vi "Configure Sample Rate [ARB].vi"(8 "error in (no error)":errorcluster, 9 "sample rate (1000 Samp/s)":dbl[unit]=1000.0 format="%^.2e", 11 "CS++Fgen in":refnum<class "CS++Fgen.lvclass">) -> (0 "error out":errorcluster, 3 "CS++Fgen out":refnum<class "CS++Fgen.lvclass">)   [LabVIEW 2013, in "CS++Fgen.lvlib" / "CS++Fgen.lvclass"]
doc: "This VI configures the rate at which the function generator produces the points that make up arbitrary waveforms. When you configure the function generator to produce an arbitrary sequence, this is the sample rate for all arbitrary waveforms in the sequence.\n \nNotes:\n\n(1) This VI is part of the IviFgenArbWfm [ARB] extension group."
uses:
  CS++Fgen.lvclass
  Core/Classes/CS++ProcessVariables/ProcessVariable/PV.lvclass
  Core/Classes/CS++ProcessVariables/ProcessVariable/PV.lvclass/PV.ctl
  CS++Fgen.lvclass/CS++Fgen.ctl
  Core/Classes/CS++ProcessVariables/PVConnection/PVConnection.lvclass
  Core/Classes/CS++ProcessVariables/ProcessVariable/Write Data.vi
  Core/Classes/CS++ProcessVariables/ProcessVariable/Write Timestamp.vi
  Core/Classes/CS++ProcessVariables/ProcessVariable/Write Quality.vi
  Core/Classes/CS++ProcessVariables/ProcessVariable/Write status.vi
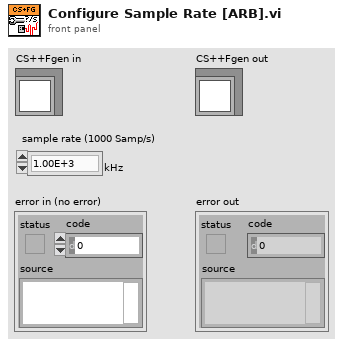
[diagram p1: front panel]
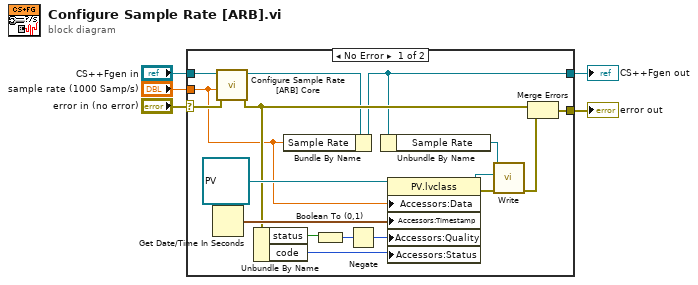
[diagram p0: block diagram]
diagram:
  n1 = case shown="No Error" "error in (no error)" {
    selector: "error in (no error)" -> [w21 w24]
    tunnel: [w10 w24] -> w4
    tunnel: [w6 w23] -> w2
    tunnel: "CS++Fgen in" -> [w22 w23]
    tunnel: "sample rate (1000 Samp/s)" -> [w8 _]
    frame No Error {
      n2 = Get Date/Time In Seconds() -> (seconds since 1Jan1904=w20:timestamp)
      n3 = call-dynamic "Configure Sample Rate [ARB] Core.vi"("error in (no error)"=w21, "sample rate (1000 Samp/s)"=w8, "CS++Fgen in"=w22) -> ("error out"=w9:errorcluster, "CS++Fgen out"=w7:refnum<class "CS++Fgen.lvclass">)  [unwired: 7 in]
      n4 = Unbundle By Name(w9) -> ("status"=w15:bool, "code"=w13:i32)
      n5 = Bundle By Name(cluster=w7, "Sample Rate"=w8) -> (w6:refnum<class "CS++Fgen.lvclass">)
      n6 = Boolean To (0,1)(Boolean=w15) -> (0, 1=w14:i16)
      n7 = Negate(x=w14) -> (-x=w12:i16)
      n8 = Unbundle By Name(w6) -> ("Sample Rate"=w11:refnum<class "PVConnection.lvclass">)
      n9 = property class="PV.lvclass"(reference=refnum<class "PV.lvclass"> refnum ("PV"), "Accessors:Data"=w8, "Accessors:Timestamp"=w20, "Accessors:Quality"=w12, "Accessors:Status"=w13) -> (reference out=w17:refnum<class "PV.lvclass">, error out=w18:errorcluster)  [unwired: 1 in]
      n10 = call-dynamic "Write.vi"("error in (no error)"=w18, "PV"=w17, "PVConnection in"=w11) -> ("error out"=w16:errorcluster)  [unwired: 7 in, 1 out]
      n11 = Merge Errors(w9, w16) -> (w10:errorcluster)
    }
    frame Error {
    }
  }
  "error out" <- w4
  "CS++Fgen out" <- w2
